vi "MatchFiducial.vi"(8 "error in":errorcluster, 9 "Image In":T2, 10 "Template Image":T2) -> (0 "error out":errorcluster, 1 "Y (um)":dbl format="%#_4g", 2 "X (um)":dbl format="%#_4g", 3 "Image Out":T2, 4 "Angle":sgl, 5 "Number of Matches":i32)   [LabVIEW 2018]
uses:
  <vilib>/vision/Image Controls.llb/IMAQ Image.ctl
  <vilib>/vision/NI_Vision_Development_Module.lvlib
panel:
  in  "Settings":T1={"Algorithm"=2, "Number of Matches Requested"=1, "Minimum Match Score"=400.0, "SubPixel Accuracy"=TRUE, "Rotation Angle Ranges"=[{"Start"=0.0, "End"=360.0}], "Show Search Area"=TRUE, "Show Result"=TRUE} {"Algorithm" items=["All", "Low Discrepancy Sampling", "Grayscale Value Pyramid", "Gradients Pyramid"]}
  in  "Range":cluster{"Lower value":sgl, "Upper value":sgl}={"Lower value"=128.0, "Upper value"=255.0} {"Upper value" format="%.2f"; "Lower value" format="%.2f"}
  out "Image Dst Out":T2(plugin-control)
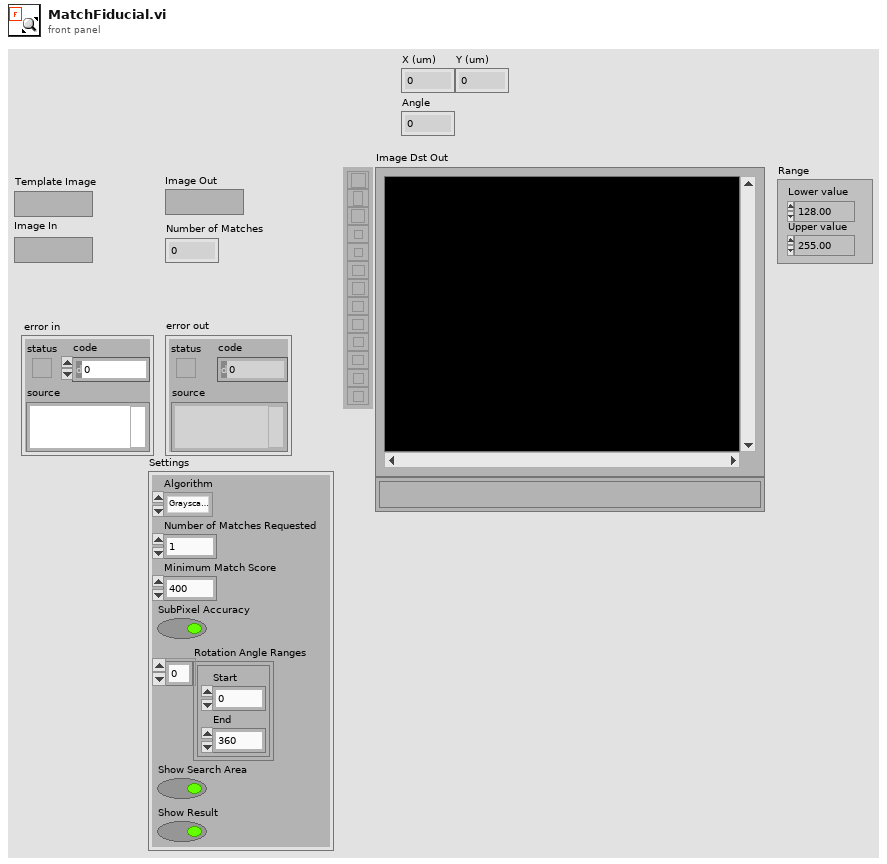
[diagram p1: front panel]
types:
  T1 = cluster{"Algorithm":i32, "Number of Matches Requested":i32, "Minimum Match Score":sgl, "SubPixel Accuracy":bool, "Rotation Angle Ranges":cluster{"Start":sgl, "End":sgl}[], "Show Search Area":bool, "Show Result":bool}
  T2 = typedef "IMAQ Image.ctl" = refnum<image>
  T3 = typedef "IMAQ Rectangle" = cluster{"Left":i32, "Top":i32, "Right":i32, "Bottom":i32, "Rotation":dbl}
  T4 = cluster{"Position":cluster{"x":sgl, "y":sgl}, "Angle":sgl, "Scale":sgl, "Score":sgl, "Bounding Box":cluster{"x":sgl, "y":sgl}[]}[]
  T5 = cluster{"Position":cluster{"x":sgl, "y":sgl}, "Angle":sgl, "Scale":sgl, "Score":sgl, "Bounding Box":cluster{"x":sgl, "y":sgl}[]}
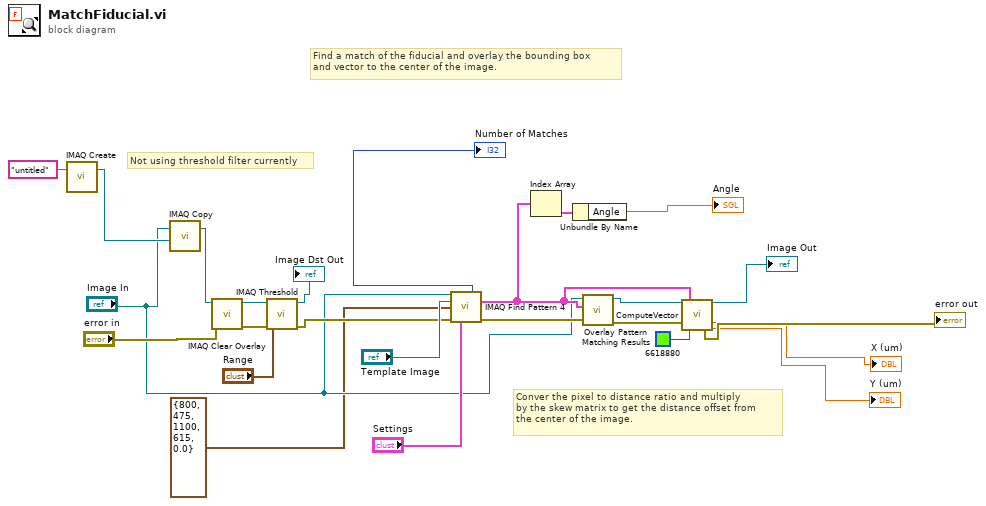
[diagram p0: block diagram]
diagram:
  # "Conver the pixel to distance ratio and multiply \nby the skew matrix to get the distance offset from \nthe center of the image."
  # "Not using threshold filter currently"
  # "Find a match of the fiducial and overlay the bounding box\nand vector to the center of the image."
  n1 = call "IMAQ Create"("Image Name"="untitled") -> ("New Image"=w10:T2)  [unwired: 4 in, 1 out]
  n2 = call "IMAQ Copy"("Image Dst"=w10, "Image Src"="Image In") -> ("Image Dst Out"=w9:T2)  [unwired: 4 in, 1 out]
  n3 = call "IMAQ Clear Overlay"("error in (no error)"="error in", "Image"=w9) -> ("error out"=w14:errorcluster, "Image Out"=w12:T2)  [unwired: 8 in]
  n4 = call "IMAQ Threshold"("error in (no error)"=w14, "Range"="Range", "Image Src"=w12) -> ("error out"=w13:errorcluster, "Image Dst Out"=→"Image Dst Out":T2)  [unwired: 7 in]
  n5 = call "IMAQ Find Pattern 4"("Image"="Image In", "Template"="Template Image", "Search Rect"=T3 {"Left"=800, "Top"=475, "Right"=1100, "Bottom"=615, "Rotation"=0.0}, "error in"=w13, "Settings"="Settings") -> ("Number of Matches"=→"Number of Matches":i32, "Matches (pixel)"=w20:T4, "error out"=w25:errorcluster)  [unwired: 4 in, 4 out]
  n6 = Index Array(array=w20) -> (element=w19:T5)  [unwired: 1 in]
  n7 = Unbundle By Name(w19) -> ("Angle"=→"Angle":sgl)
  n8 = call "Overlay Pattern Matching Results.vi"("error in"=w25, "Matches"=w20, "Image"="Image In") -> ("error out"=w24:errorcluster, "Image Out"=w23:T2)  [unwired: 7 in]
  n9 = call "ComputeVector.vi"("Image"=w23, "error in"=w24, "Matches"=w20, "Color"=u32 6618880) -> ("error out"=→"error out":errorcluster, "Image Out"=→"Image Out":T2, "X (um)"=→"X (um)":dbl, "Y (um)"=→"Y (um)":dbl)  [unwired: 10 in, 2 out]
